vi "HFRR ADV v017 new software.vi"() -> ()   [LabVIEW 2025] (continued)
              frame True {
                n4003 = Increment(x=w4777) -> (x+1=w4776:dbl)
                "T cycle" <- w4776
                n4004 = local write "Json St Flg"(FALSE ("Json St Flg")) -> ()
              }
            }
          }
          frame Enabled {
          }
        }
        n4005 = local read "Quit"() -> (w4759:bool)
      }
    }
    frame Enabled {
    }
  }
  n4006 = stacked-sequence {
    tunnel: [w5157] -> w39
    frame #0 {
      w5157 = FALSE ("Upload \nConfirmed")
      n4007 = local write "Upload \nConfirmed"(w5157) -> ()
      n4008 = local write "St Str"("") -> ()
    }
  }
  n4009 = disable-structure shown="Disabled" {
    disable-tunnel: w39 -> [w5158 _]
    frame Disabled {
      n4010 = case shown="True" {
        selector: _ -> [_ _]
        tunnel: w5158 -> [_ w5159]
        frame False {
        }
        frame True {
          n4011 = while {
            tunnel: [w5165] -> _
            tunnel: w5159 -> [_]
            i -> [w5165]
            stop <- w5160 stop-if-true
            n4012 = local read "Json End Flg"() -> (w5164:bool)
            n4013 = Wait (ms)(milliseconds to wait=u32 20 ("Refresh Rate (ms)")) -> ()  [unwired: 1 out]
            n4014 = local read "refresh flag"() -> (w5161:bool)
            n4015 = local read "RUN"() -> (w5162:bool)
            n4016 = And(x=w5162, y=w5161) -> (x .and. y?=w5163:bool)
            n4017 = Or(x=w5163, y=w5164) -> (x .or. y?=w5166:bool)
            "AR Led" <- w5166
            n4018 = case shown="True" w5166 {
              frame False {
              }
              frame True {
                w5183 = "\",\""
                n4019 = local read "UUID"() -> (w5181:string)
                n4020 = local write "refresh flag"(FALSE ("refresh flag")) -> ()
                n4021 = local read "time"() -> (w5170:dbl)
                n4022 = Multiply(x=w5170, y=60.0) -> (x*y=w5169:dbl)
                n4023 = Concatenate Strings("UUID\" : \"", w5181, "\"}") -> (w5184:string)
                n4024 = Number To Fractional String(number=w5169, width (-)=i16 10, precision (6)=i16 4) -> (F-format string=w5198:string)  [unwired: 1 in]
                n4025 = Concatenate Strings("{", "\"Time\":\"", w5198, w5183) -> (w5193:string)
                n4026 = stacked-sequence {
                  tunnel: w5183 -> [w5246 w5254 w5261 w5269 w5277 w5286 w5293]
                  tunnel: [w5247 _ _ _ _ _ _] -> w5197
                  tunnel: [_ w5255 _ _ _ _ _] -> w5196
                  tunnel: [_ _ w5262 _ _ _ _] -> w5195
                  tunnel: [_ _ _ w5271 _ _ _] -> w5194
                  tunnel: w5184 -> [_ _ _ _ _ _ w5304]
                  tunnel: [_ _ _ _ _ _ w5303] -> w5180
                  tunnel: [_ _ _ _ _ w5283 _] -> w5179
                  tunnel: [_ _ _ _ w5276 _ _] -> w5178
                  frame #0 {
                    n4027 = local read "NORMAL LOAD"() -> (w5245:dbl)
                    n4028 = Number To Fractional String(number=w5245, width (-)=i16 10, precision (6)=i16 4) -> (F-format string=w5248:string)  [unwired: 1 in]
                    n4029 = Concatenate Strings("NormalLoad\":\"", w5248, w5246) -> (w5247:string)
                  }
                  frame #1 {
                    n4030 = local read "Temp"() -> (w5253:dbl)
                    n4031 = Number To Fractional String(number=w5253, width (-)=i16 10, precision (6)=i16 4) -> (F-format string=w5256:string)  [unwired: 1 in]
                    n4032 = Concatenate Strings("Temperature\":\"", w5256, w5254) -> (w5255:string)
                  }
                  frame #2 {
                    n4033 = local read "cof"() -> (w5259:dbl)
                    n4034 = Number To Fractional String(number=w5259, width (-)=i16 10, precision (6)=i16 4) -> (F-format string=w5263:string)  [unwired: 1 in]
                    n4035 = Concatenate Strings("FrictionalForce\":\"", w5263, w5261) -> (w5262:string)
                  }
                  frame #3 {
                    n4036 = local read "Set Hz"() -> (w5267:dbl)
                    n4037 = Multiply(x=w5267, y=60.0) -> (x*y=w5266:dbl)
                    n4038 = Number To Fractional String(number=w5266, width (-)=i16 10, precision (6)=i16 4) -> (F-format string=w5272:string)  [unwired: 1 in]
                    n4039 = Concatenate Strings("Speed\":\"", w5272, w5269) -> (w5271:string)
                  }
                  frame #4 {
                    n4040 = local read item#-1() -> (w5275)
                    n4041 = Number To Fractional String(number=w5275, width (-)=i16 10, precision (6)=i16 4) -> (F-format string=w5279:string)  [unwired: 1 in]
                    n4042 = Concatenate Strings("LinearDeformation\":\"", w5279, w5277) -> (w5276:string)
                  }
                  frame #5 {
                    n4043 = local read "AIR TEMP"() -> (w5282:dbl)
                    n4044 = local read "Json St Flg"() -> (w5284:bool)
                    n4045 = local read "Json End Flg"() -> (w5285:bool)
                    n4046 = Number To Fractional String(number=w5282, width (-)=i16 10, precision (6)=i16 4) -> (F-format string=w5288:string)  [unwired: 1 in]
                    n4047 = Concatenate Strings("Vibration\":\"", w5288, w5286) -> (w5283:string)
                    n4048 = And(x=w5284, y=w5285) -> ()  [unwired: 1 out]
                  }
                  frame #6 {
                    n4049 = local read "Json End Flg"() -> (w5292:bool)
                    n4050 = Get Date/Time In Seconds() -> (seconds since 1Jan1904=w5300:timestamp)
                    n4051 = local read "Json St Flg"() -> (w5291:bool)
                    n4052 = To Double Precision Float(number=w5300) -> (double precision float=w5299:dbl)
                    n4053 = Subtract(x=w5299, y=2082844800.0) -> (x-y=w5297:dbl)
                    n4054 = Number To Fractional String(number=w5297, width (-)=i16 12, precision (6)=i16 0) -> (F-format string=w5294:string)  [unwired: 1 in]
                    n4055 = case shown="True" w5292 {
                      tunnel: ["" w5307] -> w5301
                      tunnel: w5294 -> [_ w5308]
                      tunnel: w5293 -> [_ w5306]
                      frame False {
                      }
                      frame True {
                        n4056 = local write "Json End Flg"(FALSE ("Json St Flg")) -> ()
                        n4057 = Concatenate Strings("End\": \"", w5308, w5306) -> (w5307:string)
                      }
                    }
                    n4058 = case shown="True" w5291 {
                      tunnel: [w5311 w5314] -> w5302
                      tunnel: w5294 -> [_ w5315]
                      tunnel: w5293 -> [_ w5312]
                      frame False {
                        n4059 = local read "St Str"() -> (w5311:string)
                      }
                      frame True {
                        n4060 = Concatenate Strings("Start\":\"", w5315, w5312) -> (w5314:string)
                        "St Str" <- w5314
                        n4061 = local write "Json St Flg"(FALSE ("Json St Flg")) -> ()
                      }
                    }
                    n4062 = Concatenate Strings(w5302, w5301, w5304) -> (w5303:string)
                  }
                }
                n4063 = local read "FILE"() -> (w5172:string)
                n4064 = Concatenate Strings("\",\"OperatorID\":\"" ("string"), "Operator ID") -> (w5175:string)
                n4065 = Concatenate Strings("\",\"DatasetTitle\":\"" ("string"), w5172) -> (w5174:string)
                n4066 = Concatenate Strings("\",\"SerialNumber\":\"" ("string"), "Serial No") -> (w5204:string)
                n4067 = Concatenate Strings("\",\"ModelNumber\":\"" ("string"), "Model No") -> (w5203:string)
                n4068 = Concatenate Strings(w5204, w5203) -> (w5186:string)
                n4069 = Concatenate Strings("{\"SecretKey\":\"", "Secret Key", w5186, w5175, w5174, "\",\"Samples\":[") -> (w5191:string)
                n4070 = Concatenate Strings(w5193, w5197, w5196, w5195, w5194, w5178, w5179, w5180) -> (w5192:string)
                n4071 = Concatenate Strings(w5191, w5192, "]}") -> (w5190:string)
                n4072 = stacked-sequence {
                  tunnel: w5190 -> [w5219 _ _]
                  tunnel: [_ _ w5236] -> _
                  frame #0 {
                    (unwired) FALSE ("convert eol (F)")
                    w5221 = enum16{"start", "end", "current"}."start" ("pos mode (0:2)")
                    n4073 = Path To String(path="Path") -> (string=w5227:string)
                    n4074 = Concatenate Strings(w5227, "\\", "Data File Name") -> (w5229:string)
                    n4075 = local write "standard output"(" ") -> ()
                    n4076 = String To Path(string=w5229) -> (path=w5218:path)
                    n4077 = call <vilib>:"Open_Create_Replace File.vi"("advisory dialog? (display:T)"=FALSE, "function (open:0)"=T32."create or replace", "file path"=w5218) -> ("error out"=w5232:errorcluster, "refnum"=w5231:refnum<file>)  [unwired: 5 in, 2 out]
                    n4078 = Set File Position(refnum=w5231, from (0:start)=w5221, error in=w5232) -> (refnum out=w5212:refnum<file>, error out=w5211:errorcluster)  [unwired: 1 in]
                    n4079 = Write to Binary File(file (use dialog)=w5212, data=" ", error in=w5211, 5:FALSE ("prepend array or string size? (T)")) -> (refnum out=w5222:refnum<file>, error out=w5223:errorcluster)  [unwired: 2 in, 1 out]
                    n4080 = Set File Position(offset (in bytes) (0)=w5221, refnum=w5222, error in=w5223) -> (refnum out=w5215:refnum<file>, error out=w5214:errorcluster)  [unwired: 1 in]
                    n4081 = Write to Binary File(file (use dialog)=w5215, data=w5219, error in=w5214, 5:FALSE ("prepend array or string size? (T)")) -> (error out=w5217:errorcluster)  [unwired: 2 in, 2 out]
                    n4082 = flat-sequence {
                      tunnel: w5218 -> [w5234]
                      tunnel: w5217 -> [_]
                      frame #0 {
                        n4083 = call <vilib>:"Read Characters From File.vi"("file path (dialog if empty)"=w5234) -> ("character string"=→"JSON string":string)  [unwired: 5 in, 3 out]
                      }
                    }
                    "SinglePoint" <- w5219
                  }
                  frame #1 {
                  }
                  frame #2 {
                    (unwired) "\"Stored\": true" ("string")
                    n4084 = call <vilib>:"System Exec.vi"("run minimized? (F)"=TRUE, "wait until completion? (T)"=TRUE, "working directory"=path "C:/LAB-IQ-NXT", "command line"="C:\\LAB-IQ-NXT\\JPost.bat") -> ("standard error"=→"Respose From Server":string, "standard output"=w5239:string)  [unwired: 4 in, 2 out]
                    "standard output" <- w5239
                    n4085 = Match Pattern(string=w5239, regular expression="JSON Check String") -> (match substring=w5237:string, offset past match=w5236:i32)  [unwired: 1 in, 2 out]
                    n4086 = Equal?(x=w5237, y="JSON Check String") -> (x = y?=→"Upload \nConfirmed":bool)
                  }
                }
              }
            }
            n4087 = local read "Quit"() -> (w5160:bool)
          }
        }
      }
    }
    frame Enabled {
    }
  }
  n4088 = disable-structure shown="Disabled" {
    disable-tunnel: _ -> [w5322 _]
    frame Disabled {
      n4089 = while {
        shift-right: [w5330] -> w5318
        shift-left: _ -> [w5331]
        shift-right: [w5328] -> w5319
        shift-left: errorcluster {"status"=TRUE, "code"=0, "source"="Init"} ("error out") -> [w5329]
        shift-right: [w5326] -> _
        shift-left: "" -> [w5327]
        tunnel: [w5324] -> _
        tunnel: w5322 -> [_]
        i -> [w5324]
        stop <- w5323 stop-if-true
        n4090 = flat-sequence {
          tunnel: [w5332] -> w5325
          frame #0 {
            n4091 = Wait (ms)(milliseconds to wait=10.0 ("Delay")) -> (millisecond timer value=w5332:u32)
          }
        }
        n4092 = case shown="No Error" w5329 {
          selector: w5329 -> [w5362 w5481]
          tunnel: [w5345 w5483] -> w5330
          tunnel: [w5344 w5482] -> w5328
          tunnel: w5331 -> [w5363 w5475]
          tunnel: w5327 -> [w5343 w5474]
          tunnel: [w5342 w5474] -> w5326
          tunnel: w5325 -> [_ _]
          frame No Error {
            n4093 = Concatenate Strings("\r", "\n") -> (w5354:string)  [unwired: 1 in]
            n4094 = case shown="True" w5355 {
              tunnel: w5363 -> [w5387 w5394]
              tunnel: w5362 -> [w5386 w5393]
              tunnel: [w5387 w5392] -> w5361
              tunnel: [w5386 w5391] -> w5341
              tunnel: w5354 -> [_ w5390]
              frame False {
              }
              frame True {
                n4095 = VISA Write(VISA resource name=w5394, write buffer=w5390, error in (no error)=w5393) -> (VISA resource name out=w5392:refnum<visa-resource-name>, error out=w5391:errorcluster)  [unwired: 1 out]
                n4096 = local write "Read String"("") -> ()
                n4097 = local write item#-1(FALSE) -> ()
              }
            }
            n4098 = property class="Instr"(reference=w5361, error in=w5341) -> (reference out=w5360:refnum<visa-resource-name>, error out=w5359:errorcluster, "Serial Settings:Number of Bytes at Serial Port"=w5358:u32)
            n4099 = Greater?(x=w5358, y=u32 100) -> (0:w5356:bool)
            n4100 = case shown="True" w5356 {
              tunnel: w5360 -> [w5397 w5421]
              tunnel: w5359 -> [w5396 w5420]
              tunnel: w5358 -> [_ w5419]
              tunnel: [w5397 w5418] -> w5347
              tunnel: [w5396 w5417] -> w5346
              tunnel: w5343 -> [w5395 w5416]
              tunnel: [w5395 ""] -> w5342
              frame False {
              }
              frame True {
                w5406 = u32 6 ("y")
                # "Page 84 of \nmanual"
                n4101 = VISA Read(VISA resource name=w5421, byte count=w5419, error in (no error)=w5420) -> (VISA resource name out=w5418:refnum<visa-resource-name>, read buffer=w5414:string, error out=w5417:errorcluster)  [unwired: 1 out]
                n4102 = while {
                  tunnel: w5414 -> [w5470]
                  tunnel: [w5466] -> w5408 mode=indexing
                  tunnel: [w5460] -> w5412 mode=indexing
                  tunnel: [w5458] -> _
                  i -> [w5458]
                  stop <- w5463 stop-if-true
                  n4103 = String Subset(string=w5470, offset (0)=w5458) -> (substring=w5465:string)  [unwired: 1 in]
                  n4104 = String To Byte Array(string=w5465) -> (unsigned byte array=w5469:u8[])
                  n4105 = String Length(string=w5465) -> (length=w5464:i32)
                  n4106 = Index Array(array=w5469) -> (element=w5468:u8)  [unwired: 1 in]
                  n4107 = Equal To 0?(x=w5464) -> (x = 0?=w5463:bool)
                  n4108 = Number To Boolean Array(number=w5468) -> (Boolean array=w5462:bool[])
                  n4109 = Reverse 1D Array(array=w5462) -> (reversed array=w5461:bool[])
                  n4110 = And(x=w5462, y=bool[] [FALSE, FALSE, FALSE, FALSE, FALSE, FALSE, TRUE, TRUE] ("Boolean array")) -> (x .and. y?=w5466:bool[])
                  n4111 = And(x=w5461, y=bool[] [FALSE, FALSE, TRUE, TRUE, TRUE, TRUE, TRUE, TRUE] ("Boolean array")) -> (x .and. y?=w5460:bool[])
                }
                n4112 = Concatenate Strings(w5416, w5414) -> (→"Read String":string)
                n4113 = while {
                  tunnel: w5408 -> [w5457] mode=indexing
                  tunnel: [w5453] -> w5411
                  i -> [w5453]
                  stop <- w5454 stop-if-true
                  n4114 = Search 1D Array(1D array=w5457, element=TRUE) -> (index of element=w5455:i32)  [unwired: 1 in]
                  n4115 = Less Than 0?(x=w5455) -> (x < 0?=w5454:bool)
                }
                n4116 = Delete From Array(array=w5412, length=w5411, index (row)=0) -> (array with subset deleted=w5407:bool[][])  [unwired: 1 in, 1 out]
                n4117 = Array Size(array=w5407) -> (size(s)=w5409:i32[])
                n4118 = Index Array(array=w5409) -> (element=w5401:i32)  [unwired: 1 in]
                n4119 = Greater?(x=w5401, y=w5406) -> (0:w5404:bool)
                n4120 = Subtract(x=w5401, y=w5406) -> (x-y=w5405:u32)
                n4121 = Select(t=w5405, s=w5404, f=u32 0) -> (s? t:f=w5402:u32)
                n4122 = while {
                  tunnel: w5407 -> [w5440]
                  tunnel: [w5442] -> w5400 mode=indexing
                  tunnel: w5402 -> [w5424]
                  i -> [w5441]
                  stop <- w5439 stop-if-true
                  w5431 = 6 ("index")
                  w5430 = 2 ("length")
                  # "Page 65 of \nmanual"
                  n4123 = Multiply(x=u32 3 ("y"), y=w5441) -> (x*y=w5438:u32)
                  n4124 = Divide(x=u32 102 ("y"), y=u32 65520) -> (x/y=w5448:dbl)
                  n4125 = Greater Or Equal?(x=w5438, y=w5424) -> (x >= y?=w5439:bool)
                  n4126 = Index Array(array=w5440, index (row) #1=w5438) -> (element #1=w5436:bool[], element #2=w5435:bool[], element #3=w5434:bool[])  [unwired: 5 in]
                  n4127 = Reverse 1D Array(array=w5436) -> (reversed array=w5429:bool[])
                  n4128 = Reverse 1D Array(array=w5435) -> (reversed array=w5433:bool[])
                  n4129 = Reverse 1D Array(array=w5434) -> (reversed array=w5432:bool[])
                  n4130 = Delete From Array(array=w5429, length=w5430, index=w5431) -> (array with subset deleted=w5425:bool[])  [unwired: 1 out]
                  n4131 = Delete From Array(array=w5433, length=w5430, index=w5431) -> (array with subset deleted=w5426:bool[])  [unwired: 1 out]
                  n4132 = Delete From Array(array=w5432, length=w5430, index=w5431) -> (array with subset deleted=w5427:bool[])  [unwired: 1 out]
                  n4133 = Insert Into Array(array=bool[] [] ("Boolean array"), new element #1=w5425, new element #2=w5426, new element #3=w5427) -> (w5428:bool[])  [unwired: 1 in]
                  n4134 = Boolean Array To Number(Boolean array=w5428) -> (number=w5437:u32)
                  n4135 = Multiply(x=w5448, y=w5437) -> (x*y=w5447:dbl)
                  n4136 = Decrement(x=w5447) -> (x-1=w5446:dbl)
                  n4137 = Divide(x=w5446, y=u32 100) -> (x/y=w5444:dbl)
                  n4138 = Multiply(x=w5444, y=u32 10) -> (x*y=w5442:dbl)
                }
                n4139 = Delete From Array(array=w5400) -> (array with subset deleted=w5399:dbl[])  [unwired: 2 in, 1 out]
                "Waveform Graph 5" <- w5399
                "Waveform Chart 3" <- w5399
                n4140 = call-poly <vilib>:"Mean.vi"("X"=w5399) -> ("mean"=w5398:dbl)  [unwired: 1 out]
                n4141 = case shown="True" {
                  selector: _ -> [_ _]
                  tunnel: w5398 -> [_ w5423]
                  frame False {
                  }
                  frame True {
                    n4142 = local write item#-1(FALSE ("Zero 4")) -> ()
                    "z_measure" <- w5423
                  }
                }
              }
            }
            n4143 = local read item#-1() -> (w5338)
            n4144 = local read item#-1() -> (w5337)
            n4145 = local read item#-1() -> (w5339)
            n4146 = local read item#-1() -> (w5336)
            n4147 = case shown="True" w5334 {
              tunnel: w5338 -> [_ w5366]
              tunnel: w5339 -> [_ w5365]
              frame False {
              }
              frame True {
                n4148 = Build Array(w5366, w5365) -> (w5364:void[])
                n4149 = local read item#-1() -> (w5369)
                n4150 = Build Array (concatenate)(w5369, w5364) -> (w5367:void[])
                n4151 = local write item#-1(w5367) -> ()
                n4152 = local write item#-1(FALSE ("Boolean 8")) -> ()
              }
            }
            n4153 = call "Build XY Graph"("Enable"=w5336, "Reset"=w5337, "Y Input"=w5339, "X Input"=w5338) -> ("XY Graph"=w5335:cluster{"Y":dbl[], "Y":dbl[]}[])  [unwired: 6 in, 1 out]
            n4154 = case shown="True" {
              selector: _ -> [_ _]
              frame False {
              }
              frame True {
                n4155 = local read item#-1() -> (w5370)
                n4156 = Index Array(array=w5370, index (col) #1=0 ("disabled index (col)"), index (col) #2=1 ("index (col)")) -> (element #1=w5372, element #2=w5371)  [unwired: 2 in]
                n4157 = call <vilib>:"Linear Fit.vi"("Y"=w5372, "X"=w5371) -> ()  [unwired: 9 in, 5 out]
                n4158 = local write item#-1(FALSE ("Boolean 9")) -> ()
              }
            }
            n4159 = case shown="True" {
              selector: _ -> [_ _]
              frame False {
              }
              frame True {
                n4160 = local write item#-1(dbl[][] [] ("Captured Values")) -> ()
                n4161 = local write item#-1(FALSE ("Boolean 7")) -> ()
              }
            }
            n4162 = Concatenate Strings("\r", "\n") -> (w5349:string, w5348:string)
            n4163 = case shown="True" w5340 {
              tunnel: w5347 -> [w5379 w5385]
              tunnel: w5346 -> [w5378 w5384]
              tunnel: [w5379 w5383] -> w5345
              tunnel: [w5378 w5382] -> w5344
              tunnel: w5349 -> [_ w5381]
              frame False {
              }
              frame True {
                n4164 = VISA Write(VISA resource name=w5385, write buffer=w5381, error in (no error)=w5384) -> (VISA resource name out=w5383:refnum<visa-resource-name>, error out=w5382:errorcluster)  [unwired: 1 out]
                n4165 = local write item#-1(FALSE ("WRITE")) -> ()
              }
            }
          }
          frame Error {
            w5473 = u16 10 items=["1.0"=10, "1.5"=15, "2.0"=20] ("stop bits (10: 1 bit)")
            n4166 = Wait (ms)(milliseconds to wait=u32 20) -> ()  [unwired: 1 out]
            n4167 = VISA Close(VISA resource name=w5475, error in (no error)=w5481) -> (error out=w5480:errorcluster)
            n4168 = call <vilib>:"Clear Errors.vi"("error in (no error)"=w5480) -> ("error out"=w5479:errorcluster)  [unwired: 5 in, 1 out]
            n4169 = call-poly "VISA Configure Serial Port"("timeout (10sec)"=u32 200, "Enable Termination\nChar (T)"=TRUE ("Enable Termination\nChar (T)"), "baud rate (9600)"=u32 921600, "error in (no error)"=w5479, "stop bits (10: 1 bit)"=w5473) -> ("VISA resource name"=w5471:refnum<visa-resource-name>, "VISA resource name out"=w5483:refnum<visa-resource-name>, "error out"=w5482:errorcluster)  [unwired: 8 in]
          }
        }
        n4170 = local read "Quit"() -> (w5323:bool)
      }
      n4171 = VISA Close(VISA resource name=w5318, error in (no error)=w5319) -> (error out=w5317:errorcluster)
      n4172 = call <vilib>:"Clear Errors.vi"("error in (no error)"=w5317) -> ()  [unwired: 5 in, 2 out]
    }
    frame Enabled {
    }
  }
  n4173 = disable-structure shown="Disabled" {
    disable-tunnel: _ -> [w5488 _]
    frame Disabled {
      n4174 = while {
        tunnel: [w5495] -> _
        shift-right: [w5492] -> w5485
        shift-left: _ -> [w5494]
        shift-right: [w5493] -> w5486
        shift-left: errorcluster {"status"=TRUE, "code"=0, "source"="Init"} ("error out") -> [w5491]
        tunnel: w5488 -> [_]
        i -> [w5495]
        stop <- w5489 stop-if-true
        n4175 = flat-sequence {
          tunnel: w5491 -> [w5586]
          tunnel: [w5586] -> w5490
          frame #0 {
            n4176 = Wait (ms)(milliseconds to wait=u32 50) -> ()  [unwired: 1 out]
          }
        }
        n4177 = case shown="No Error" w5490 {
          selector: w5490 -> [w5536 w5579]
          tunnel: w5494 -> [w5535 w5578]
          tunnel: [w5502 w5569] -> w5493
          tunnel: [w5503 w5577] -> w5492
          frame No Error {
            w5529 = T33 {"Mode"=enum."RTU", "Slave Address"=1} ("Serial Parameters")
            n4178 = call-poly <vilib>:"MB Serial Master Query (poly).vi"("VISA resource name"=w5535, "Starting Address"=i16 1000, "Quantity"=u16 1, "Timeout"=u32 1000, "error in"=w5536, "Serial Parameters"=w5529) -> ("VISA resource name out"=w5530:refnum<visa-resource-name>, "Input Registers"=w5532:u16[], "error out"=w5528:errorcluster)  [unwired: 10 in, 1 out]
            n4179 = Random Number (0-1)() -> (number: 0 to 1=w5517:dbl)
            n4180 = Index Array(array=w5532, index=0) -> (element=w5527:u16)
            n4181 = Subtract(x=w5517, y=0.5) -> (x-y=w5516:dbl)
            n4182 = Divide(x=w5527, y=10 ("index")) -> (x/y=w5521:dbl)
            n4183 = Multiply(x=w5516, y=0.5) -> (x*y=w5515:dbl)
            n4184 = Add(x=w5521, y=w5515) -> (x+y=w5520:dbl)
            n4185 = local read "Amb temp"() -> (w5504:dbl)
            n4186 = Multiply(x=w5520, y=0.2) -> (x*y=w5524:dbl)
            n4187 = Multiply(x=w5504, y=0.8) -> (x*y=w5522:dbl)
            n4188 = Add(x=w5524, y=w5522) -> (x+y=w5505:dbl)
            n4189 = local read "set temp old"() -> (w5499:dbl)
            n4190 = local write "Amb temp"(w5505) -> ()
            n4191 = Select(t="SetTemp 2", s="Heater", f=100.0) -> (s? t:f=w5500:dbl)
            n4192 = Not Equal?(x=w5500, y=w5499) -> (x != y?=w5498:bool)
            n4193 = case shown="True" w5498 {
              tunnel: w5530 -> [w5564 w5566]
              tunnel: [w5563 w5566] -> w5510
              tunnel: w5528 -> [w5562 w5565]
              tunnel: [w5561 w5565] -> w5508
              tunnel: w5500 -> [w5556 _]
              tunnel: w5529 -> [w5558 w5567]
              tunnel: [w5558 w5567] -> w5511
              frame True {
                n4194 = Multiply(x=w5556, y=10 ("index")) -> (x*y=w5555:dbl)
                n4195 = call-poly <vilib>:"MB Serial Master Query (poly).vi"("VISA resource name"=w5564, "Address"=u16 0, "Holding Register"=w5555, "Timeout"=u32 1000, "error in"=w5562, "Serial Parameters"=w5558) -> ("VISA resource name out"=w5563:refnum<visa-resource-name>, "error out"=w5561:errorcluster)  [unwired: 11 in, 1 out]
                "set temp old" <- w5556
              }
              frame False {
              }
            }
            n4196 = flat-sequence {
              tunnel: [w5537] -> _
              tunnel: [w5537] -> w5507
              tunnel: w5508 -> [w5537]
              frame #0 {
                n4197 = Wait (ms)(milliseconds to wait=u32 100) -> ()  [unwired: 1 out]
              }
            }
            n4198 = call "Elapsed Time12"("Time Target (s)"=2.0, "Auto Reset"=TRUE) -> ("Time has Elapsed"=w5512:bool)  [unwired: 10 in, 7 out]
            n4199 = case shown="True" w5512 {
              tunnel: w5511 -> [w5541 w5554]
              tunnel: [w5541 w5554] -> _
              tunnel: [w5540 w5552] -> w5503
              tunnel: w5510 -> [w5540 w5553]
              tunnel: [w5539 w5550] -> w5502
              tunnel: w5507 -> [w5539 w5551]
              frame False {
              }
              frame True {
                n4200 = call-poly <vilib>:"MB Serial Master Query (poly).vi"("VISA resource name"=w5553, "Starting Address"=i16 1003 ("Addr"), "Quantity"=u16 1, "Timeout"=u32 1000, "error in"=w5551, "Serial Parameters"=w5554) -> ("VISA resource name out"=w5552:refnum<visa-resource-name>, "Input Registers"=w5547:u16[], "error out"=w5550:errorcluster)  [unwired: 10 in, 1 out]
                n4201 = Index Array(array=w5547, index=0) -> (element=w5546:u16)
                n4202 = Divide(x=w5546, y=u16 10) -> (x/y=w5542:dbl)
                n4203 = local write "set temp old"(w5542) -> ()
                n4204 = local write "SetTemp"(w5542) -> ()
              }
            }
            "Error Code" <- w5502
            n4205 = Unbundle(w5502) -> ("status"=→"TK4 status":bool)  [unwired: 2 out]
            "SetTemp" <- "SetTemp 2"
          }
          frame Error {
            w5581 = u16 0 items=["None", "Odd", "Even", "Mark", "Space"] ("Parity")
            w5582 = u16 0 items=["None", "XON/XOFF", "RTS/CTS", "XON/XOFF & RTS/CTS", "DTR/DSR", "XON/XOFF & DTR/DSR"] ("Flow Control")
            n4206 = VISA Clear(VISA resource name=w5578, error in (no error)=w5579) -> (VISA resource name out=w5572:refnum<visa-resource-name>, error out=w5570:errorcluster)
            n4207 = VISA Close(VISA resource name=w5572, error in (no error)=w5570) -> (error out=w5571:errorcluster)
            n4208 = call <vilib>:"Clear Errors.vi"("error in (no error)"=w5571) -> ("error out"=w5580:errorcluster)  [unwired: 5 in, 1 out]
            n4209 = Unbundle By Name(T33 {"Mode"=enum."RTU", "Slave Address"=1} ("input cluster")) -> ("Mode"=w5583:enum16{"RTU", "ASCII"})
            n4210 = call <vilib>:"MB Serial Init.vi"("Timeout"=u32 100, "Flow Control"=w5582, "Mode"=w5583, "error in (no error)"=w5580, "Parity"=w5581, "Baud Rate"=u32 9600, "VISA resource name"="Lubrication System COM Port :") -> ("error out"=w5569:errorcluster, "VISA resource name out"=w5577:refnum<visa-resource-name>)  [unwired: 3 in]
            n4211 = local write "set temp old"(0.0 ("set temp old")) -> ()
            n4212 = Unbundle(w5569) -> ("status"=w5568:bool)  [unwired: 2 out]
            n4213 = case shown="True" w5568 {
              selector: w5568 -> [_ w5585]
              frame False {
              }
              frame True {
                n4214 = local write "TK4 status"(w5585) -> ()
              }
            }
          }
        }
        n4215 = local read "Quit"() -> (w5489:bool)
      }
      n4216 = VISA Close(VISA resource name=w5485, error in (no error)=w5486) -> (error out=w5484:errorcluster)
      n4217 = call <vilib>:"Clear Errors.vi"("error in (no error)"=w5484) -> ()  [unwired: 5 in, 2 out]
    }
    frame Enabled {
    }
  }
